vi "practiceImageAnalysis - HH.vi"() -> ()   [LabVIEW 2016]
uses:
  <vilib>/vision/Image Controls.llb/IMAQ Image.ctl
  <vilib>/vision/Measure.llb/Edge Options.ctl
  <vilib>/vision/Measure.llb/Edge Polarity.ctl
  <vilib>/Analysis/NI_AALPro.lvlib
  <vilib>/Utility/file.llb/Write Delimited Spreadsheet (DBL).vi
panel:
  out "Fitted edge residue":dbl
  out "Fitted edge error":i32
  out "Fitted edge intercept":dbl
  out "Fitted edge slope":dbl
  in  "Linear fit parameter bounds":T1={"slope min"=-inf, "slope max"=inf, "intercept min"=-inf, "intercept max"=inf}
  out "x^2 fit error":i32
  out "Polynomial Coefficients":dbl[](array[numeric])
  out "Residuals":dbl[](array[numeric])
  out "Fitted SD( dI/dR )":dbl[](array[numeric])
  out "Fitted edge locations":dbl[](array[numeric])
  out "residue":dbl
  out "Fit residue vs Z":T2(graph)
  out "Fitted SD dI/dR vs Z":T3(graph)
  out "Fitted radii vs Z":T3(graph)
  out "Processing Image #":i32
  out "Derivative: Normalized Intensity vs Radius":T3(graph)
  out "Selected subarray":T4(plugin-control)
  out "Normalized Intensity vs Radius":cluster{dbl[], dbl[]}(graph)
  in  "nBins":dbl=300.0
  in  "Min":dbl
  in  "Max":dbl=300.0
  out "Fitted Circle":T5 {"Average SNR (dB)" format="%.2f"; "Average Strength" format="%.2f"; "Roundness (Real-World)" format="%.2f"; "Radius (Real-World)" format="%.2f"; "Center (Real-World)"."Y" format="%.2f"; "Center (Real-World)"."X" format="%.2f"; "Radius (Pixels)" format="%.2f"; "Center (Pixels)"."Y" format="%.2f"; "Center (Pixels)"."X" format="%.2f"}
  out "Npixel@Intensity Histogram":T6(graph)
  out "Npixel@phi Histogram":T6(graph)
  out "Npixel@R Histogram":T6(graph)
  in  "Circle ROI Descriptor":T7={"Global Rectangle"=[675, 567, 1751, 1642], "Contours"=[{"ID"=enum."External", "Type"=7, "Coordinates"=[1212, 1104, 85, 537, 0, 0]}]} {"Contours"."Type" items=["No Selection", "Point", "Line", "Rectangle", "Oval", "Polygon", "Freehand Region", "Annulus", "Unused2", "Unused3", "Broken Line", "Freehand Line", "Rotated Rectangle"]}
  in  "Circle Fit Options":T8={"Process"=enum."Get Best Edge", "Step Size"=3.0, "Max Pixel Radius"=3}
  in  "Circle Finding Options":T11={"Search  Direction"=1, "Edge Options"={"Edge Polarity"=2, "Kernel Size"=3, "Width"=3, "Minimum Edge Strength"=10.0, "Interpolation Type"=enum."Bilinear Fixed", "Data Processing Method"=enum."Average"}, "Show Search Area"=FALSE, "Show Search Lines"=FALSE, "Show Edges Found"=FALSE, "Show Result"=TRUE, "Search Area Color"=65280, "Search Lines Color"=255, "Edge Locations Color"=16776960, "Result Color"=65511, "Overlay Group Name"=""} {"Search  Direction" items=["Outside to Inside", "Inside to Outside"]; "Edge Options"."Edge Polarity" items=["All Edges", "Rising Edges", "Falling Edges"]; "Edge Options"."Minimum Edge Strength" format="%.2f"; "Edge Options"."Width" step=2; "Edge Options"."Kernel Size" step=2}
  in  "Pattern Match Settings":T12={"Algorithm"=2, "Number of Matches Requested"=1, "Minimum Match Score"=800.0, "SubPixel Accuracy"=TRUE, "Rotation Angle Ranges"=[], "Show Search Area"=FALSE, "Show Result"=TRUE} {"Rotation Angle Ranges"."End" format="%.1f"; "Rotation Angle Ranges"."Start" format="%.1f"; "Minimum Match Score" min=0 max=1000 format="%.2f"; "Number of Matches Requested" min=1; "Algorithm" items=["All", "Low Discrepancy Sampling", "Grayscale Value Pyramid", "Gradients Pyramid"]}
  out "Template Image":T4
  in  "Coordinate file for image capture":path=path "C:/Users/sciollalab/Desktop/dotCoordinates-captured.csv"
  out "Review":bool
  out "Search running?":bool
  in  "Stop and delete":bool
  out "Images Array":T4[](array[plugin-control])=["image_442_-22_00"]
  in  "error in":errorcluster
  out "error out":errorcluster
  out "Filenames Array":string[](array[string])
  in  "Naming Convention":string="image_442_-22_00.png"
  in  "Images Directory":path=path "C:/Users/sciollalab/Desktop/dots1-12-16-2016/dots_-146,-22"
  # "add linear fit to R vs Z"
  # "fit to a parabola"
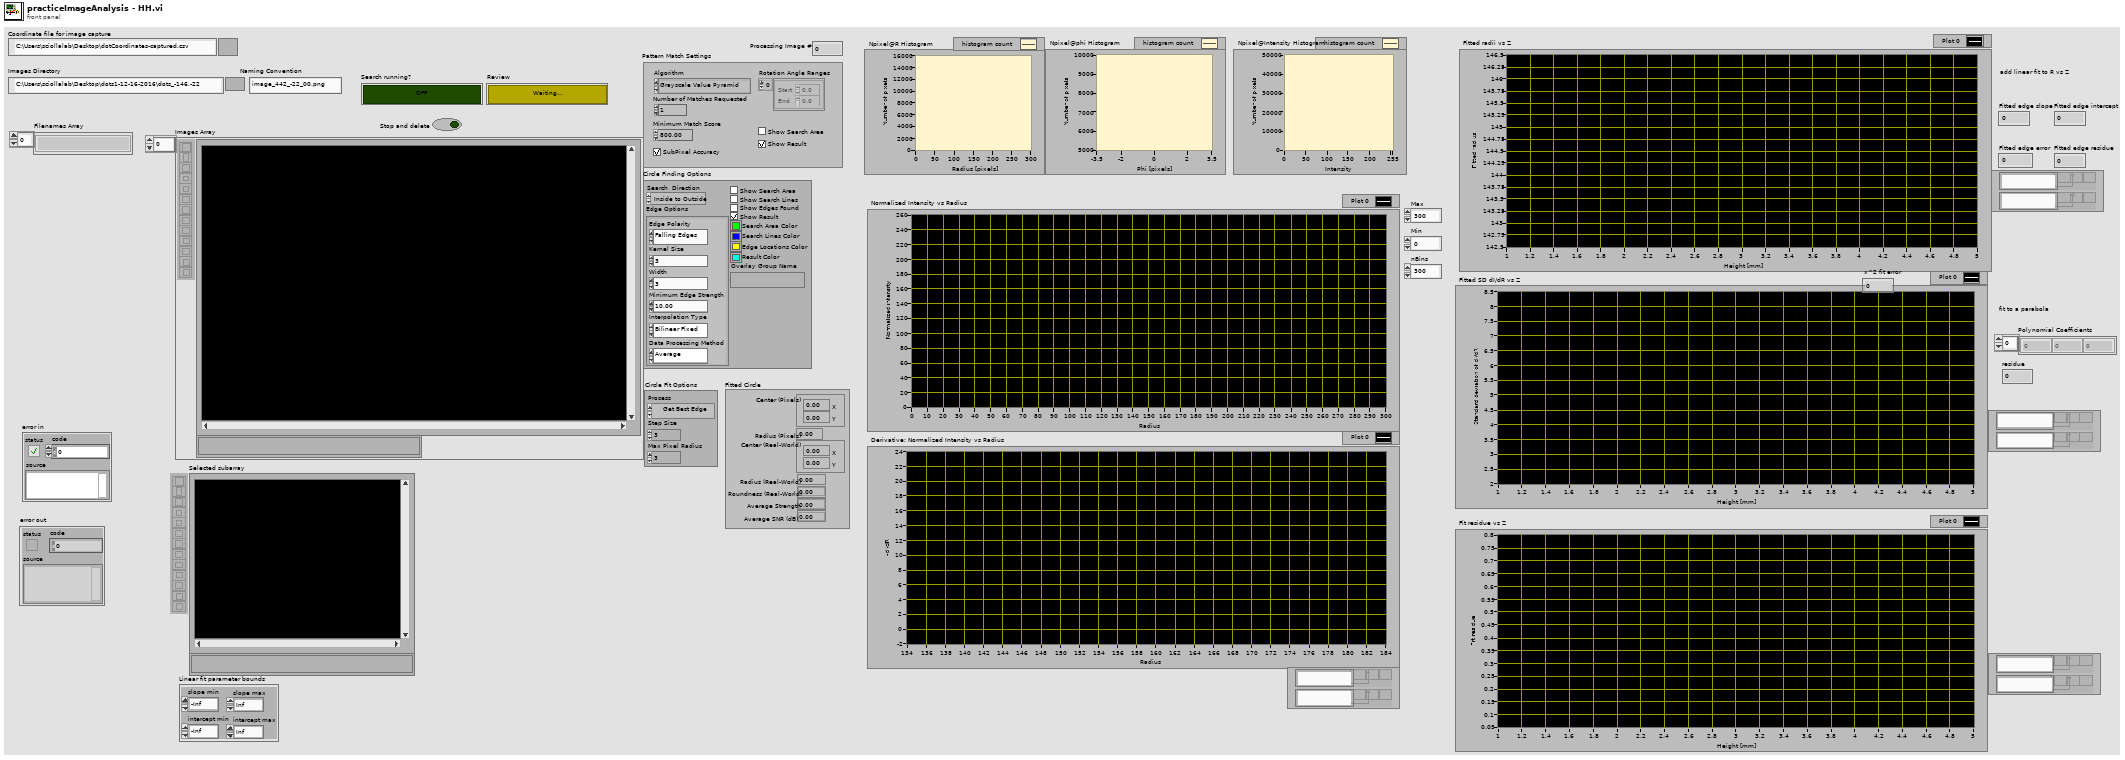
[diagram p1: front panel]
types:
  T1 = cluster{"slope min":dbl, "slope max":dbl, "intercept min":dbl, "intercept max":dbl}
  T2 = cluster{"Image coordinates in lab frame":dbl[], dbl[]}
  T3 = cluster{"Radius bins":dbl[], "Best Gaussian Fit":dbl[]}[]
  T4 = typedef "IMAQ Image.ctl" = refnum<image>
  T5 = cluster{"Center (Pixels)":cluster{"X":sgl, "Y":sgl}, "Radius (Pixels)":dbl, "Center (Real-World)":cluster{"X":sgl, "Y":sgl}, "Radius (Real-World)":dbl, "Roundness (Real-World)":dbl, "Average Strength":dbl, "Average SNR (dB)":dbl}
  T6 = cluster{"X Values":dbl[], "Histogram: h(x)":i32[]}
  T7 = cluster{"Global Rectangle":i32[], "Contours":cluster{"ID":enum32{"External", "Internal"}, "Type":u32, "Coordinates":i32[]}[]}
  T8 = cluster{"Process":enum16{"Get First Edge", "Get First + Last Edge", "Get All Edges", "Get Best Edge"}, "Step Size":dbl, "Max Pixel Radius":i32}
  T9 = typedef "Edge Options.ctl" = cluster{"Edge Polarity":T10, "Kernel Size":u32, "Width":u32, "Minimum Edge Strength":sgl, "Interpolation Type":enum32{"Zero Order", "Bilinear", "Quadratic", "Cubic", "Bilinear Fixed"}, "Data Processing Method":enum32{"Average", "Median"}}
  T10 = typedef "Edge Polarity.ctl" = u32
  T11 = cluster{"Search  Direction":u32, "Edge Options":T9, "Show Search Area":bool, "Show Search Lines":bool, "Show Edges Found":bool, "Show Result":bool, "Search Area Color":u32, "Search Lines Color":u32, "Edge Locations Color":u32, "Result Color":u32, "Overlay Group Name":string}
  T12 = cluster{"Algorithm":i32, "Number of Matches Requested":i32, "Minimum Match Score":sgl, "SubPixel Accuracy":bool, "Rotation Angle Ranges":cluster{"Start":sgl, "End":sgl}[], "Show Search Area":bool, "Show Result":bool}
  T13 = enum16{"cm", "mm", "pixels [mm/pix]", "pixels [um/pix]"}
  T14 = cluster{"initial amplitude":dbl, "initial center":dbl, "initial standard deviation":dbl, "offset":dbl}
  T15 = cluster{"Image coordinates in lab frame":dbl[], "Residuals":dbl[]}
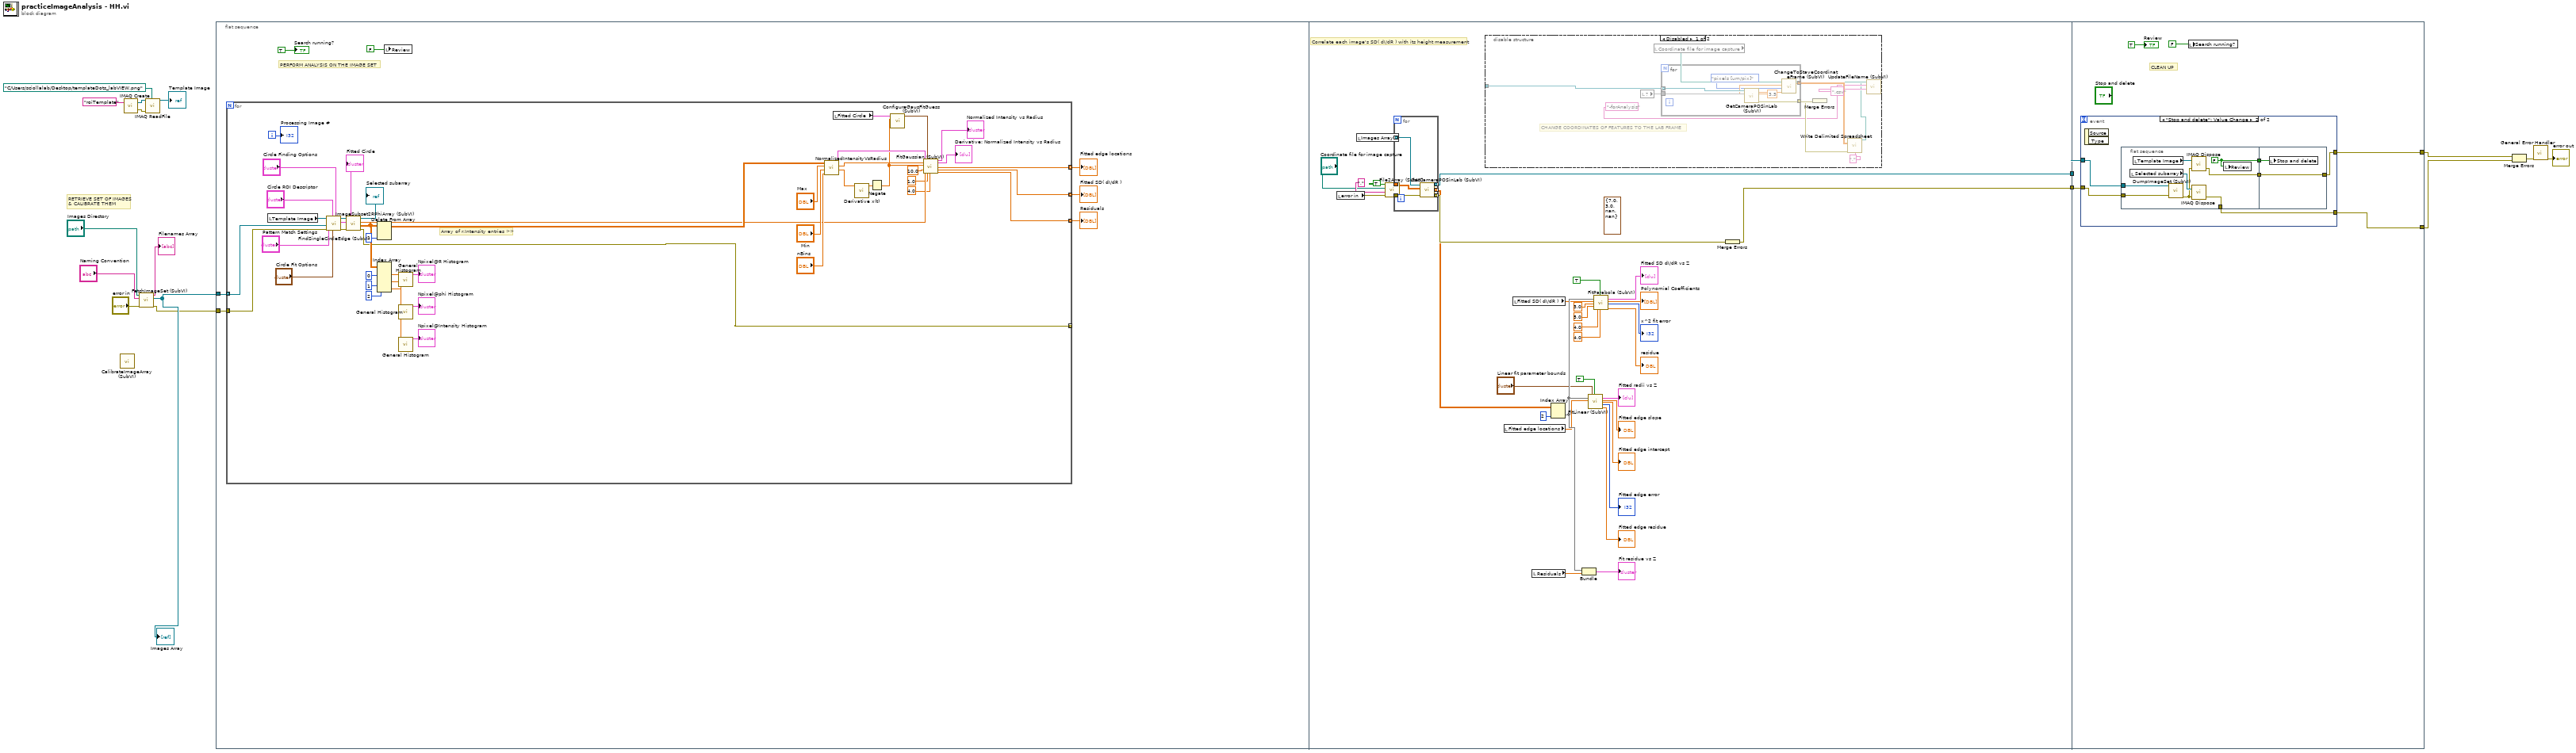
[diagram p0: block diagram]
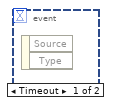
[diagram p3: hidden frame]
diagram:
  # "RETRIEVE SET OF IMAGES\n& CALIBRATE THEM"
  n1 = call "CalibrateImageArray (SubVI).vi"() -> ()  [unwired: 9 in, 2 out]
  n2 = call "IMAQ Create"("Image Name"="roiTemplate") -> ("New Image"=w7:T4, "error out"=w8:errorcluster)  [unwired: 4 in]
  n3 = call "FetchImageSet (SubVI).vi"("error in (no error)"="error in", "Naming Convention"="Naming Convention", "Images Directory"="Images Directory") -> ("error out"=w4:errorcluster, "Image Array"=w10:T4[], "Filenames Array"=→"Filenames Array":string[])  [unwired: 6 in]
  "Images Array" <- w10
  n4 = call "IMAQ ReadFile"("File Path"=path "C:/Users/sciollalab/Desktop/templateDots_labVIEW.png" ("Template File Path"), "error in (no error)"=w8, "Image"=w7) -> ("Image Out"=→"Template Image":T4)  [unwired: 4 in, 4 out]
  n5 = flat-sequence {
    tunnel: w10 -> [w22]
    tunnel: w4 -> [w21]
    tunnel: [w94] -> w3
    tunnel: [w92] -> w2
    tunnel: [w128] -> w12
    tunnel: w3 -> [w127]
    tunnel: w2 -> [w126]
    tunnel: [w125] -> w1
    frame #0 {
      # "PERFORM ANALYSIS ON THE IMAGE SET"
      n6 = for {
        tunnel: w22 -> [w67] mode=indexing
        tunnel: w21 -> [w65]
        tunnel: [w28] -> w20 mode=indexing
        tunnel: [w27] -> w19 mode=indexing
        tunnel: [w26] -> w18 mode=indexing
        tunnel: [w25] -> _ mode=indexing
        i -> [w39]
        # "Array of r,Intensity entries >>"
        n7 = local read "Template Image"() -> (w68:T4)
        n8 = call "FindSingleCircleEdge (SubVI).vi"("Circle Finding Options"="Circle Finding Options", "Circle Fit Options"="Circle Fit Options", "Circle ROI Descriptor"="Circle ROI Descriptor", "error in (no error)"=w65, "Search Image in"=w67, "Pattern Match Settings"="Pattern Match Settings", "Template in"=w68) -> ("error out"=w61:errorcluster, "Fitted Circle"=w35:T5, "Search image out"=w53:T4)  [unwired: 2 in]
        "Fitted Circle" <- w35
        n9 = call "ImageSubset2RPhiArray (SubVI).vi"("error in (no error)"=w61, "Fitted Circle"=w35, "Full Image in"=w53) -> ("error out"=w25:errorcluster, "2D Array: r, phi, intensity"=w37:dbl[][], "Radius (Pixels)"=w40:dbl, "Subset image out"=→"Selected subarray":T4)  [unwired: 5 in]
        n10 = Delete From Array(array=w37, index (col)=1 ("disabled index (col)")) -> (array with subset deleted=w49:dbl[][])  [unwired: 2 in, 1 out]
        n11 = Index Array(array=w37, index (col) #1=0 ("disabled index (col)"), index (col) #2=1 ("index (col)"), index (col) #3=2 ("index (col)")) -> (element #1=w52:dbl[], element #2=w54:dbl[], element #3=w51:dbl[])  [unwired: 3 in]
        n12 = call <vilib>:"General Histogram.vi"("X"=w52) -> ("Histogram Graph"=→"Npixel@R Histogram":T6)  [unwired: 10 in, 4 out]
        n13 = call <vilib>:"General Histogram.vi"("X"=w54) -> ("Histogram Graph"=→"Npixel@phi Histogram":T6)  [unwired: 10 in, 4 out]
        n14 = call <vilib>:"General Histogram.vi"("X"=w51) -> ("Histogram Graph"=→"Npixel@Intensity Histogram":T6)  [unwired: 10 in, 4 out]
        n15 = call "NormalizedIntensityVsRadius.vi"("nBins"="nBins", "Min"="Min", "Max"="Max", "Input Array (r,I)"=w49) -> ("Normalized Intensity"=w29:dbl[], "Radius bins"=w42:dbl[], "Normalized Intensity vs Radius"=w44:cluster{dbl[], dbl[]})  [unwired: 5 in]
        n16 = local read "Fitted Circle"() -> (w34:T5)
        n17 = call <vilib>:"Derivative x(t).vi"("X"=w29) -> ("dX/dt"=w43:dbl[])  [unwired: 9 in, 1 out]
        n18 = Negate(x=w43) -> (-x=w33:dbl[])
        n19 = call "ConfigureGausFitGuess (SubVI).vi"("Array"=w33, "Fitted Circle"=w34) -> ("initial guess out"=w36:T14)  [unwired: 9 in]
        n20 = call "FitGaussian (SubVI).vi"("Normalized Intensity vs Radius in"=w44, "x values"=w42, "y values"=w33, "Estimated mean"=w40, "Estimated width"=10.0, "initial guess"=w36, "Nsigma Low"=1.0, "Nsigma High"=4.0) -> ("data plot"=→"Normalized Intensity vs Radius":cluster{dbl[], dbl[]}, "derivative data plot with Gaussian fit"=→"Derivative: Normalized Intensity vs Radius":T3, "center"=w28:dbl, "standard deviation"=w27:dbl, "residue"=w26:dbl)  [unwired: 6 in, 1 out]
        "Processing Image #" <- w39
      }
      "Fitted edge locations" <- w20
      "Fitted SD( dI/dR )" <- w19
      "Residuals" <- w18
      n21 = local write "Review"(FALSE ("Review")) -> ()
      "Search running?" <- TRUE ("Search running?")
    }
    frame #1 {
      (unwired) T14 {"initial amplitude"=7.0, "initial center"=3.0, "initial standard deviation"=nan, "offset"=nan} ("initial guess")
      # "Correlate each image's SD( dI/dR ) with its height measurement"
      n22 = local read "error in"() -> (w101:errorcluster)
      n23 = local read "Images Array"() -> (w97:T4[])
      n24 = call "File2Array (SubVI).vi"("error in (no error) in"=w101, "File delimiter"=",", "Source array file"="Coordinate file for image capture", "Load array from file?"=TRUE) -> ("error in (no error) out"=w95:errorcluster, "Loaded array"=w96:dbl[][])  [unwired: 6 in]
      n25 = for {
        tunnel: w97 -> [w107] mode=indexing
        tunnel: w96 -> [w106]
        tunnel: w95 -> [w105]
        tunnel: [w104] -> w94 mode=indexing
        tunnel: [w103] -> w93 mode=indexing
        tunnel: [w102] -> w81 mode=indexing
        n26 = call "GetCameraPOSinLab (SubVI).vi"("error in (no error)"=w105, "Loaded array"=w106, "Refnum in"=w107) -> ("error out"=w103:errorcluster, "Image coordinates in lab frame"=w102:dbl[], "Refnum out"=w104:T4)  [unwired: 6 in]
      }
      n27 = disable-structure shown="Disabled" {
        disable-tunnel: _ -> [w109 _]
        frame Disabled {
          # "CHANGE COORDINATES OF FEATURES TO THE LAB FRAME"
          n28 = local read item#-1() -> (w117)
          n29 = local read "Coordinate file for image capture"() -> (w112:path)
          n30 = for {
            tunnel: w109 -> [w124] mode=indexing
            tunnel: w117 -> [w123]
            tunnel: [w119] -> w114 mode=concatenating
            tunnel: [w118] -> w116 mode=indexing
            n31 = call "GetCameraPOSinLab (SubVI).vi"("Loaded array"=w123, "Refnum in"=w124) -> ("error out"=w118:errorcluster, "Image coordinates in lab frame"=w122:dbl[])  [unwired: 7 in, 1 out]
            n32 = call "ChangeToStaveCoordinateFrame (SubVI).vi"("Image Origin in XYZ Stage Coords [mm]"=w122, "Units"=T13."pixels [um/pix]", "Pixel resolution"=3.5) -> ("Array (stage frame, mm)"=w119:dbl[][])  [unwired: 3 in]
          }
          n33 = Merge Errors(w116) -> (w113:errorcluster)
          n34 = call "UpdateFileName (SubVI).vi"("File Extension"=".csv" ("regular expression"), "Append to Filename"="-forAnalysis" ("name or relative path"), "Path and filename"=w112) -> ("Updated Path"=w108:path)  [unwired: 8 in]
          n35 = call-poly <vilib>:"Write Delimited Spreadsheet.vi"("file path (dialog if empty)"=w108, "2D data"=w114, "error in (no error)"=w113, "delimiter (\\t)"="," ("delimiter (\\t)")) -> ()  [unwired: 10 in, 2 out]
        }
        frame Enabled {
        }
      }
      n36 = local read "Fitted edge locations"() -> (w77:dbl[])
      n37 = local read "Fitted SD( dI/dR )"() -> (w69:dbl[])
      n38 = local read "Residuals"() -> (w84:dbl[])
      n39 = Index Array(array=w81, index (col)=2 ("disabled index (col)")) -> (element=w78:dbl[])  [unwired: 1 in]
      n40 = Bundle("Image coordinates in lab frame"=w78, "Residuals"=w84) -> (→"Fit residue vs Z":T15)  [unwired: 1 in]
      n41 = call "FitLinear (SubVI).vi"("x values"=w78, "y values"=w77, "parameter bounds"="Linear fit parameter bounds", "Use all points"=TRUE) -> ("derivative data plot with linear fit"=→"Fitted radii vs Z":T3, "slope"=→"Fitted edge slope":dbl, "intercept"=→"Fitted edge intercept":dbl, "error"=→"Fitted edge error":i32, "residue"=→"Fitted edge residue":dbl)  [unwired: 10 in, 1 out]
      n42 = call "FitParabola (SubVI).vi"("x values"=w78, "y values"=w69, "Estimated mean"=3.0 ("Radius"), "Estimated width"=5.0, "Nsigma Low"=4.0, "Use all points"=TRUE, "Nsigma High"=4.0) -> ("derivative data plot with Gaussian fit"=→"Fitted SD dI/dR vs Z":T3, "Polynomial Coefficients"=→"Polynomial Coefficients":dbl[], "error"=→"x^2 fit error":i32, "residue"=→"residue":dbl)  [unwired: 8 in, 1 out]
      n43 = Merge Errors(w93) -> (w92:errorcluster)
    }
    frame #2 {
      # "CLEAN UP"
      n44 = event shown="[1] \"Stop and delete\": Value Change" {
        selector: _ -> [_ _]
        dyn-events: _ -> [_ _]
        timeout: _ -> [_ _]
        tunnel: [_ w136] -> w128
        tunnel: w127 -> [_ w133]
        tunnel: w126 -> [_ w132]
        tunnel: [_ w131] -> w125
        event Timeout {
          n45 = event-data() -> ()  [unwired: 1 in, 2 out]
        }
        event "Stop and delete": Value Change {
          n46 = event-data() -> ()  [unwired: 1 in, 2 out]
          n47 = flat-sequence {
            tunnel: [w143] -> w135
            tunnel: [w142] -> w134
            tunnel: w133 -> [w141]
            tunnel: w132 -> [w139]
            tunnel: [w137] -> w131
            tunnel: [w146] -> w136
            tunnel: w135 -> [w146]
            tunnel: w134 -> [w145]
            frame #0 {
              w142 = FALSE ("Review")
              n48 = local read "Selected subarray"() -> (w140:T4)
              n49 = local read "Template Image"() -> (w144:T4)
              n50 = call "DumpImageSet (SubVI).vi"("error in (no error)"=w139, "Calibrated Image Array"=w141) -> ("error out"=w138:errorcluster)  [unwired: 6 in]
              n51 = call "IMAQ Dispose"("Image"=w144, "error in (no error)"=w138) -> ("error out"=w143:errorcluster)  [unwired: 4 in]
              n52 = call "IMAQ Dispose"("Image"=w140, "error in (no error)"=w138) -> ("error out"=w137:errorcluster)  [unwired: 4 in]
              n53 = local write "Review"(w142) -> ()
            }
            frame #1 {
              n54 = local write "Stop and delete"(w145) -> ()
            }
          }
        }
      }
      n55 = local write "Search running?"(FALSE ("Search running?")) -> ()
      "Review" <- TRUE ("Review")
    }
  }
  n56 = Merge Errors(w12, w1) -> (w11:errorcluster)
  n57 = call <vilib>:"General Error Handler.vi"("error in (no error)"=w11) -> ("error out"=→"error out":errorcluster)  [unwired: 10 in, 4 out]
